vi "parse load from string.vi"(8 "error in":errorcluster, 11 "message data":string) -> (0 "error out":errorcluster, 1 "target":string, 2 "engines to load":string[](array[string]), 3 "data":T1)   [LabVIEW 2013, in "module execution process.lvlib"]
uses:
  module execution process.lvlib
  <vilib>/NI/Configuration Framework/tree serializer/base file format.ctl
  <vilib>/NI/Configuration Framework/tree serializer/NISE_CEF_TreeSerializer.lvlib
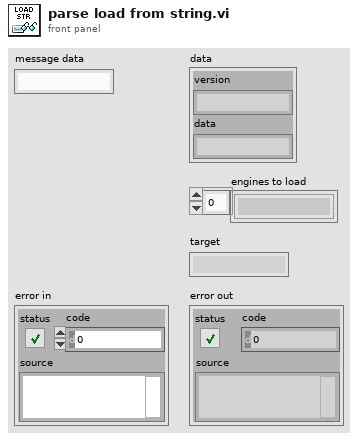
[diagram p1: front panel]
types:
  T1 = typedef "NISE_CEF_TreeSerializer.lvlib/base file format.ctl" = cluster{"version":string, "data":string}
  T2 = cluster{"data":T1, "engine to load":string[], "target to load":string}
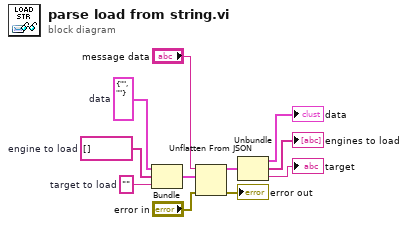
[diagram p0: block diagram]
diagram:
  w2 = ""  # target to load
  w4 = T1 {"version"="", "data"=""}  # data
  w8 = string[] []  # engine to load
  n1 = Bundle("data"=w4, "engine to load"=w8, "target to load"=w2) -> (w7:T2)  [unwired: 1 in]
  n2 = Unflatten From JSON(JSON string="message data", type and defaults=w7, error in (no error)="error in") -> (value=w6:T2, error out=→"error out":errorcluster)  [unwired: 4 in]
  n3 = Unbundle(w6) -> ("data"=→"data":T1, "engine to load"=→"engines to load":string[], "target to load"=→"target":string)
